vi "CRYReplace existing File.vi"() -> (1 "Yes or New?":bool, 3 "Replace?":bool)   [LabVIEW 2013]
panel:
  in  "dialog text":string
  in  "New":bool
  in  "Prompt":bool caption="总是取代不提示"
  in  "Yes":bool
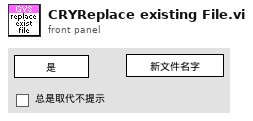
[diagram p1: front panel]
types:
  T1 = enum32{"Invalid", "Default", "Floating", "Floating/Auto-Hide", "Modal"}
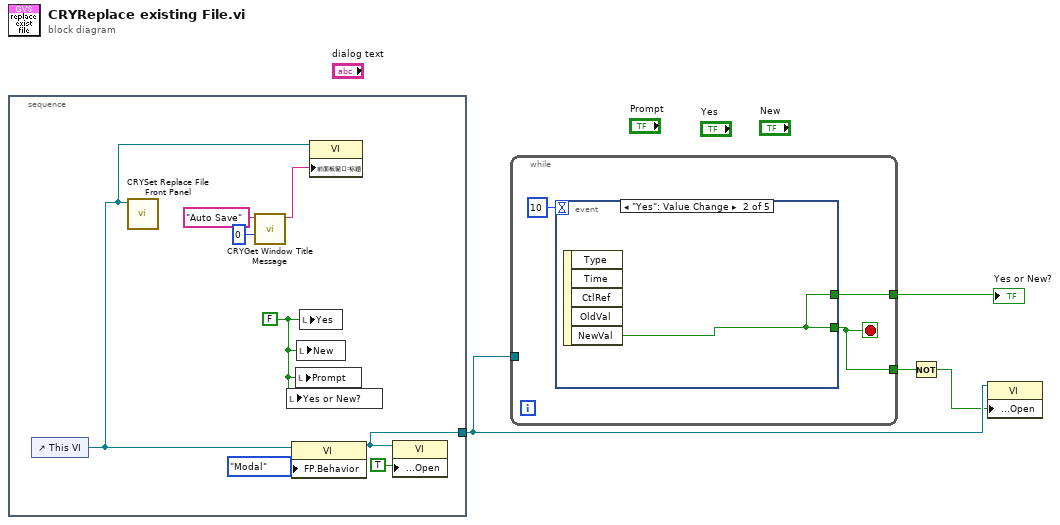
[diagram p0: block diagram]
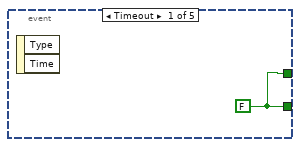
[diagram p2: hidden frame]
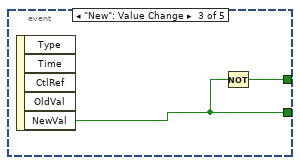
[diagram p3: hidden frame]
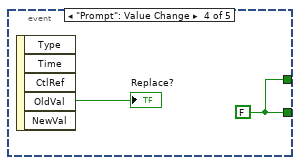
[diagram p4: hidden frame]
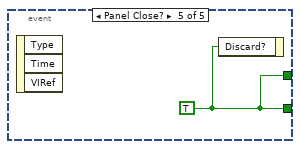
[diagram p5: hidden frame]
diagram:
  n1 = stacked-sequence {
    tunnel: [w10] -> w4
    frame #0 {
      w9 = FALSE ("Yes")
      n2 = control-ref of="This VI"() -> (w8:refnum<vi>)
      n3 = call "CRYSet Replace File Front Panel.vi"("Vi Ref"=w8) -> ()  [unwired: 11 in]
      n4 = call "CRYGet Window Title Message.vi"("No"=0, "Kind"="Auto Save") -> ("Multibyte String"=w5:string)  [unwired: 4 in, 5 out]
      n5 = local write "Yes or New?"(w9) -> ()
      n6 = property class="VI"(reference=w8, "FP.Behavior"=T1."Modal" ("Front Panel Window:Behavior")) -> (reference out=w10:refnum<vi>)  [unwired: 1 in, 1 out]
      n7 = local write "Prompt"(w9) -> ()
      n8 = local write "New"(w9) -> ()
      n9 = local write "Yes"(w9) -> ()
      n10 = property class="VI"(reference=w8, "前面板窗口:标题"=w5) -> ()  [unwired: 1 in, 2 out]
      n11 = property class="VI"(reference=w10, "Front Panel.Open"=TRUE ("Front Panel Window:Open")) -> ()  [unwired: 1 in, 2 out]
    }
  }
  n12 = while {
    tunnel: w4 -> [_]
    tunnel: [w13] -> w3
    tunnel: [w14] -> w2
    stop <- w14 stop-if-true
    n13 = event shown="[1] \"Yes\": Value Change" {
      selector: _ -> [_ _ _ _ _]
      dyn-events: _ -> [_ _ _ _ _]
      timeout: 10 -> [_ _ _ _ _]
      tunnel: [w16 w17 w19 w20 w22] -> w14
      tunnel: [w16 w17 w18 w20 w22] -> w13
      event Timeout {
        w16 = FALSE ("NewVal")
        n14 = event-data() -> ()  [unwired: 1 in, 2 out]
      }
      event "Yes": Value Change {
        n15 = event-data() -> ("NewVal"=w17:bool)  [unwired: 1 in, 4 out]
      }
      event "New": Value Change {
        n16 = event-data() -> ("NewVal"=w19:bool)  [unwired: 1 in, 4 out]
        n17 = Not(x=w19) -> (.not. x?=w18:bool)
      }
      event "Prompt": Value Change {
        w20 = FALSE ("NewVal")
        n18 = event-data() -> ("NewVal"=→"Replace?":bool)  [unwired: 1 in, 4 out]
      }
      event Panel Close? {
        w22 = TRUE ("NewVal")
        n19 = event-data() -> ()  [unwired: 1 in, 3 out]
        n20 = event-data("Discard?"=w22) -> ()  [unwired: 1 in, 1 out]
      }
    }
  }
  "Yes or New?" <- w3
  n21 = Not(x=w2) -> (.not. x?=w1:bool)
  n22 = property class="VI"(reference=w4, "Front Panel.Open"=w1) -> ()  [unwired: 1 in, 2 out]
